vi "LDC-37X4C Set Laser Current Setpoint.vi"(8 "error in (no error)":errorcluster, 10 "Current":dbl min=0.0 step=1.0, 11 "VISA resource name":refnum<visa-resource-name>) -> (0 "error out":errorcluster, 3 "VISA resource name out":refnum<visa-resource-name>)   [LabVIEW 2018]
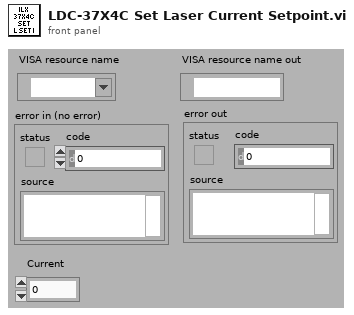
[diagram p1: front panel]
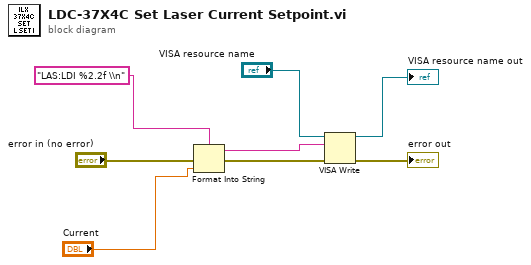
[diagram p0: block diagram]
diagram:
  n1 = Format Into String(format string="LAS:LDI %2.2f \\n", error in="error in (no error)", "Current") -> (resulting string=w7:string, error out=w5:errorcluster)  [unwired: 1 in]
  n2 = VISA Write(VISA resource name="VISA resource name", write buffer=w7, error in (no error)=w5) -> (VISA resource name out=→"VISA resource name out":refnum<visa-resource-name>, error out=→"error out":errorcluster)  [unwired: 1 out]
